vi "LabVIEW DataType to Message Element DataType.vi"(8 "error in":errorcluster, 11 "type":T2) -> (0 "error out":errorcluster, 1 "Supported?":bool, 2 "Array?":bool, 3 "MessageElementType":T1)   [LabVIEW 2019, in "grpc-lvsupport.lvlib"]
uses:
  grpc-lvsupport.lvlib
  <vilib>/Utility/Data Type/Type Definitions/Data Type.ctl
  Message Element Type.ctl
  <vilib>/Utility/Data Type/NI_Data Type.lvlib
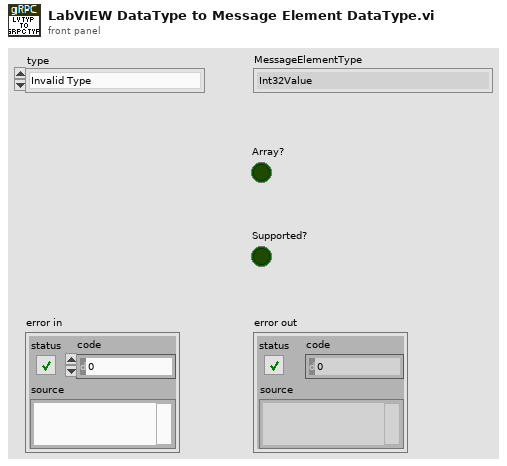
[diagram p1: front panel]
types:
  T1 = typedef "grpc-lvsupport.lvlib/Message Element Type.ctl" = enum32{"Int32Value", "FloatValue", "DoubleValue", "BoolValue", "StringValue", "MessageValue", "Int64Value", "UInt32Value", "UInt64Value", "EnumValue", "Bytes", "Fixed64", "Fixed32", "SFixed64", "SFixed32", "SInt64", "SInt32"}
  T2 = typedef "NI_Data Type.lvlib/Data Type.ctl" = enum8{"Invalid Type", "Void", "I8", "I16", "I32", "I64", "U8", "U16", "U32", "U64", "Single Float", "Double Float", "Extended Float", "Single Complex", "Double Complex", "Extended Complex", "Enum U8", "Enum U16", "Enum U32", "Enum U64", "Single Float With Unit", "Double Float With Unit", "Extended Float With Unit", "Single Complex with Unit", "Double Complex with Unit", "Extended Complex with Unit", "Boolean", "String", "Path", "Picture", "Tag", "Array", "Cluster", "Variant", "LV Variant", "Waveform", "Timestamp", "Digital Waveform", "Digital Data", "ExpressData", "Refnum", "External Data", "VI", "Poly VI", "LabVIEW Class Instance", "Fixed Point", "Set Collection", "Map Collection"}
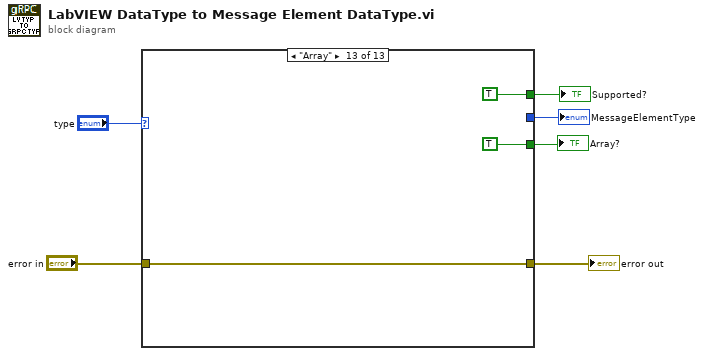
[diagram p0: block diagram]
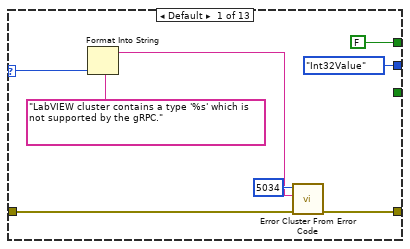
[diagram p2: hidden frame]
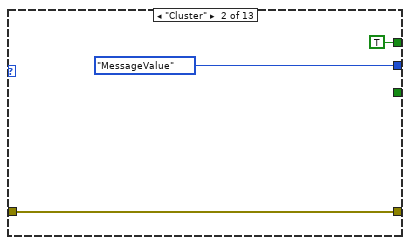
[diagram p3: hidden frame]
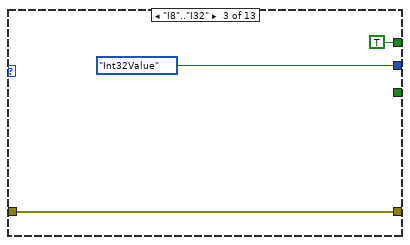
[diagram p4: hidden frame]
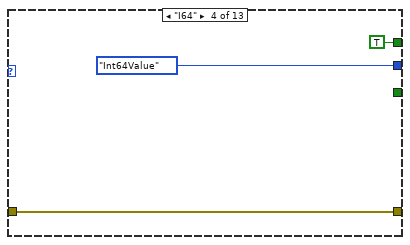
[diagram p5: hidden frame]
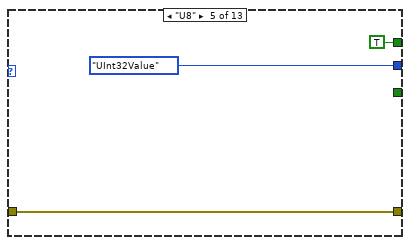
[diagram p6: hidden frame]
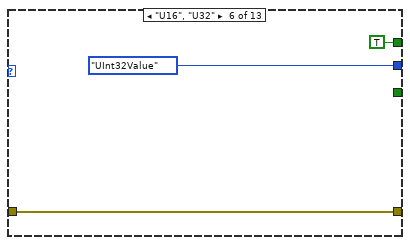
[diagram p7: hidden frame]
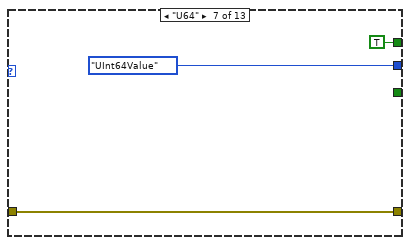
[diagram p8: hidden frame]
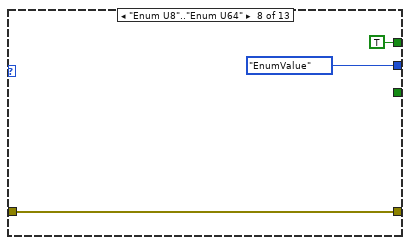
[diagram p9: hidden frame]
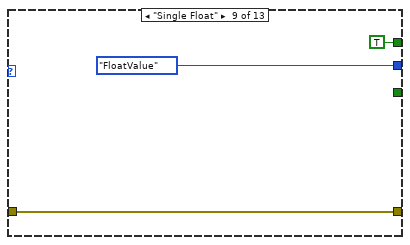
[diagram p10: hidden frame]
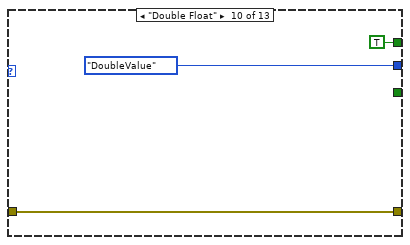
[diagram p11: hidden frame]
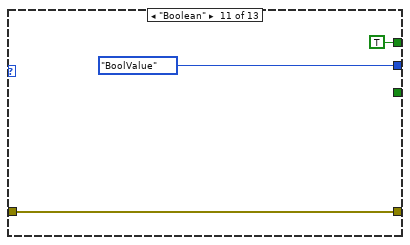
[diagram p12: hidden frame]
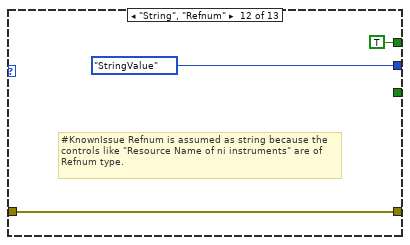
[diagram p13: hidden frame]
diagram:
  n1 = case shown="\"Array\"" "type" {
    selector: "type" -> [w10 _ _ _ _ _ _ _ _ _ _ _ _]
    tunnel: [Message_Element_Type."Int32Value" ("MessageElementType") Message_Element_Type."MessageValue" ("MessageElementType") Message_Element_Type."Int32Value" ("MessageElementType") Message_Element_Type."Int64Value" ("MessageElementType") Message_Element_Type."UInt32Value" ("MessageElementType") Message_Element_Type."UInt32Value" ("MessageElementType") Message_Element_Type."UInt64Value" ("MessageElementType") Message_Element_Type."EnumValue" ("MessageElementType") Message_Element_Type."FloatValue" ("MessageElementType") Message_Element_Type."DoubleValue" ("MessageElementType") Message_Element_Type."BoolValue" ("MessageElementType") Message_Element_Type."StringValue" ("MessageElementType") _] -> w3
    tunnel: [FALSE TRUE TRUE TRUE TRUE TRUE TRUE TRUE TRUE TRUE TRUE TRUE TRUE] -> w2
    tunnel: [_ _ _ _ _ _ _ _ _ _ _ _ TRUE] -> w1
    tunnel: "error in" -> [w7 w17 w20 w23 w26 w29 w32 w35 w38 w41 w44 w47 w50]
    tunnel: [w14 w17 w20 w23 w26 w29 w32 w35 w38 w41 w44 w47 w50] -> w5
    frame Default {
      n2 = Format Into String(format string="LabVIEW cluster contains a type '%s' which is not supported by the gRPC.", w10) -> (resulting string=w8:string)  [unwired: 2 in, 1 out]
      n3 = call <vilib>:"Error Cluster From Error Code.vi"("error in (no error)"=w7, "error message (\"\")"=w8, "error code (0)"=5034) -> ("error out"=w14:errorcluster)  [unwired: 6 in]
    }
    frame "Cluster" {
    }
    frame "I8".."I32" {
    }
    frame "I64" {
    }
    frame "U8" {
    }
    frame "U16", "U32" {
    }
    frame "U64" {
    }
    frame "Enum U8".."Enum U64" {
    }
    frame "Single Float" {
    }
    frame "Double Float" {
    }
    frame "Boolean" {
    }
    frame "String", "Refnum" {
      # "#KnownIssue Refnum is assumed as string because the controls like \"Resource Name of ni instruments\" are of Refnum type."
    }
    frame "Array" {
    }
  }
  "MessageElementType" <- w3
  "Supported?" <- w2
  "Array?" <- w1
  "error out" <- w5
